vi "UMLEditor RemoveStaticObjects.vi"(5 "error in (no error)":errorcluster) -> (19 "error out":errorcluster)   [LabVIEW 2012]
uses:
  <resource>/Framework/Providers/Open_GDS/UML/StateDiagramGraph_class/StateDiagramGraph.lvclass
  <resource>/Framework/Providers/Open_GDS/UML/UseCaseDiagramGraph_class/UseCaseDiagramGraph.lvclass
  <resource>/Framework/Providers/Open_GDS/UML/SequenceDiagramGraph_class/SequenceDiagramGraph.lvclass
  <resource>/Framework/Providers/Open_GDS/UML/ClassDiagramGraph_class/ClassDiagramGraph.lvclass
  <resource>/Framework/Providers/Open_GDS/UML/AbstractEdge_class/AbstractEdge.lvclass
  <resource>/Framework/Providers/Open_GDS/UML/AbstractNode_class/AbstractNode.lvclass
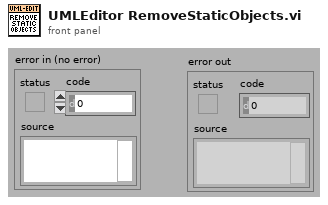
[diagram p1: front panel]
types:
  T1 = typedef "ClassDiagramGraph.lvclass/ClassAttributes.ctl" = cluster{"Base class":T2}
  T2 = typedef "Graph.lvclass/ClassAttributes.ctl" = cluster{"NODE_PROT":refnum<class "AbstractNode.lvclass">[], "NodeNames":string[], "EDGE_PROT":refnum<class "AbstractEdge.lvclass">[], "EdgeNames":string[]}
  T3 = typedef "SequenceDiagramGraph.lvclass/ClassAttributes.ctl" = cluster{"Base class":T2}
  T4 = typedef "UseCaseDiagramGraph.lvclass/ClassAttributes.ctl" = cluster{"Base class":T2}
  T5 = typedef "StateDiagramGraph.lvclass/ClassAttributes.ctl" = cluster{"Base class":T2}
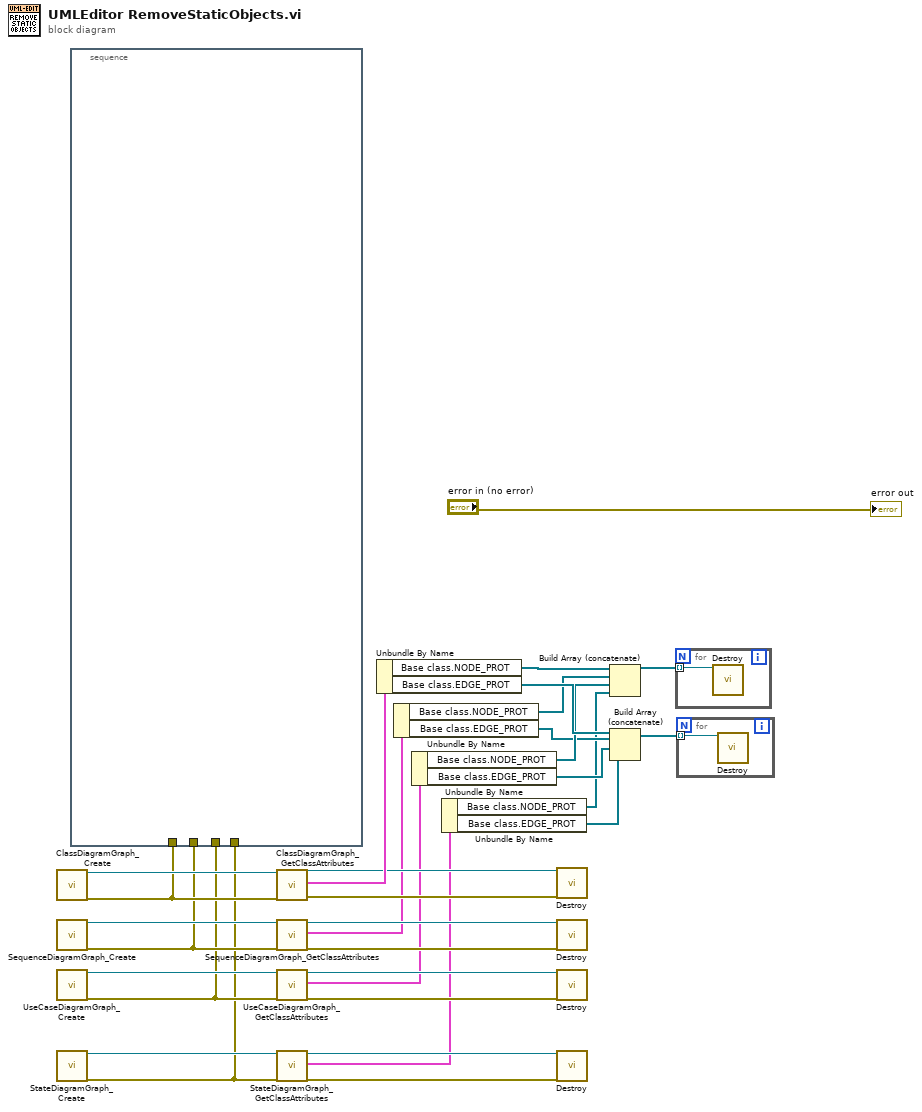
[diagram p0: block diagram]
diagram:
  n1 = call <resource>:"ClassDiagramGraph_Create.vi"() -> ("reference out"=w30:refnum<class "ClassDiagramGraph.lvclass">, "error out"=w10:errorcluster)  [unwired: 3 in, 15 out]
  n2 = call <resource>:"SequenceDiagramGraph_Create.vi"() -> ("reference out"=w22:refnum<class "SequenceDiagramGraph.lvclass">, "error out"=w9:errorcluster)  [unwired: 3 in, 15 out]
  n3 = call <resource>:"UseCaseDiagramGraph_Create.vi"() -> ("reference out"=w21:refnum<class "UseCaseDiagramGraph.lvclass">, "error out"=w8:errorcluster)  [unwired: 3 in, 15 out]
  n4 = call <resource>:"StateDiagramGraph_Create.vi"() -> ("reference out"=w5:refnum<class "StateDiagramGraph.lvclass">, "error out"=w4:errorcluster)  [unwired: 4 in, 14 out]
  n5 = stacked-sequence {
    tunnel: w10 -> [_]
    tunnel: w9 -> [_]
    tunnel: w8 -> [_]
    tunnel: w4 -> [_]
    frame #0 {
    }
  }
  n6 = call <resource>:"ClassDiagramGraph_GetClassAttributes.vi"("reference in"=w30, "error in (no error)"=w10) -> ("reference out"=w28:refnum<class "ClassDiagramGraph.lvclass">, "Class attributes out"=w29:T1, "error out"=w27:errorcluster)  [unwired: 15 out]
  n7 = call <resource>:"SequenceDiagramGraph_GetClassAttributes.vi"("reference in"=w22, "error in (no error)"=w9) -> ("reference out"=w20:refnum<class "SequenceDiagramGraph.lvclass">, "Class attributes out"=w16:T3, "error out"=w19:errorcluster)  [unwired: 15 out]
  n8 = call <resource>:"UseCaseDiagramGraph_GetClassAttributes.vi"("reference in"=w21, "error in (no error)"=w8) -> ("reference out"=w18:refnum<class "UseCaseDiagramGraph.lvclass">, "Class attributes out"=w15:T4, "error out"=w17:errorcluster)  [unwired: 15 out]
  n9 = call <resource>:"StateDiagramGraph_GetClassAttributes.vi"("reference in"=w5, "error in (no error)"=w4) -> ("reference out"=w6:refnum<class "StateDiagramGraph.lvclass">, "Class attributes out"=w3:T5, "error out"=w7:errorcluster)  [unwired: 15 out]
  n10 = Unbundle By Name(w29) -> ("Base class.NODE_PROT"=w26:refnum<class "AbstractNode.lvclass">[], "Base class.EDGE_PROT"=w24:refnum<class "AbstractEdge.lvclass">[])
  n11 = Unbundle By Name(w16) -> ("Base class.NODE_PROT"=w14:refnum<class "AbstractNode.lvclass">[], "Base class.EDGE_PROT"=w12:refnum<class "AbstractEdge.lvclass">[])
  n12 = Unbundle By Name(w15) -> ("Base class.NODE_PROT"=w13:refnum<class "AbstractNode.lvclass">[], "Base class.EDGE_PROT"=w11:refnum<class "AbstractEdge.lvclass">[])
  n13 = Unbundle By Name(w3) -> ("Base class.NODE_PROT"=w2:refnum<class "AbstractNode.lvclass">[], "Base class.EDGE_PROT"=w1:refnum<class "AbstractEdge.lvclass">[])
  n14 = call-dynamic "Destroy.vi"("reference"=w28, "error in (no error)"=w27) -> ()  [unwired: 16 in, 2 out]
  n15 = call-dynamic "Destroy.vi"("reference"=w20, "error in (no error)"=w19) -> ()  [unwired: 16 in, 2 out]
  n16 = call-dynamic "Destroy.vi"("reference"=w18, "error in (no error)"=w17) -> ()  [unwired: 16 in, 2 out]
  n17 = call-dynamic "Destroy.vi"("reference"=w6, "error in (no error)"=w7) -> ()  [unwired: 16 in, 2 out]
  n18 = Build Array (concatenate)(w26, w14, w13, w2) -> (w25:refnum<class "AbstractNode.lvclass">[])
  n19 = Build Array (concatenate)(w24, w12, w11, w1) -> (w23:refnum<class "AbstractEdge.lvclass">[])
  n20 = for {
    tunnel: w25 -> [w32] mode=indexing
    n21 = call-dynamic "Destroy.vi"("reference"=w32) -> ()  [unwired: 17 in, 2 out]
  }
  n22 = for {
    tunnel: w23 -> [w33] mode=indexing
    n23 = call-dynamic "Destroy.vi"("reference"=w33) -> ()  [unwired: 17 in, 2 out]
  }
  "error out" <- "error in (no error)"
